vi "weightSerialRead_LoadCell_Fixed_S.vi"(9 "VISA resource name":refnum<visa-resource-name>="COM5") -> (1 "Boolean":bool=TRUE, 2 "Current Weight":string)   [LabVIEW 2019]
uses:
  Program Files (x86)/National Instruments/LabVIEW 2019/examples/Instrument IO/Serial/support/Serial - Settings.ctl
  Program Files (x86)/National Instruments/LabVIEW 2019/examples/Instrument IO/Serial/support/Serial - XON-XOFF Characters.ctl
  Program Files (x86)/National Instruments/LabVIEW 2019/examples/Instrument IO/Serial/support/Serial - ASCII Characters.ctl
  <vilib>/Instr/_visa.llb/VISA Configure Serial Port (Instr).vi
panel:
  in  "Termination Character":u8=10 format="%.0x"
  in  "End Write on Termination Character?":bool=TRUE
  in  "XON/XOFF Characters":T1={"XON"=enum."DC1", "XOFF"=enum."DC3"}
  in  "Serial Settings":T3={"baud rate"=9600, "data bits"=8, "parity"=enum."None", "stop bits"=10, "flow control"=0} {"flow control" items=["None"=0, "XON/XOFF"=1, "RTS/CTS"=2, "DTR/DSR"=4]; "stop bits" items=["1.0"=10, "1.5"=15, "2.0"=20]; "data bits" min=5 max=8 step=1; "baud rate" items=["75"=75, "110"=110, "134"=134, "150"=150, "300"=300, "600"=600, "1200"=1200, "1800"=1800, "2400"=2400, "4800"=4800, "7200"=7200, "9600"=9600, "14400"=14400, "19200"=19200, "28800"=28800, "38400"=38400, "56000"=56000, "57600"=57600, "115200"=115200, "128000"=128000, "230400"=230400]}
  in  "End Read on Termination Character?":bool=TRUE
  in  "Read Count":u32=1000
  out "number":dbl
  in  "Command":string="*IDN?"
  in  "Read":bool=TRUE
  in  "Stop":bool
  in  "Write":bool
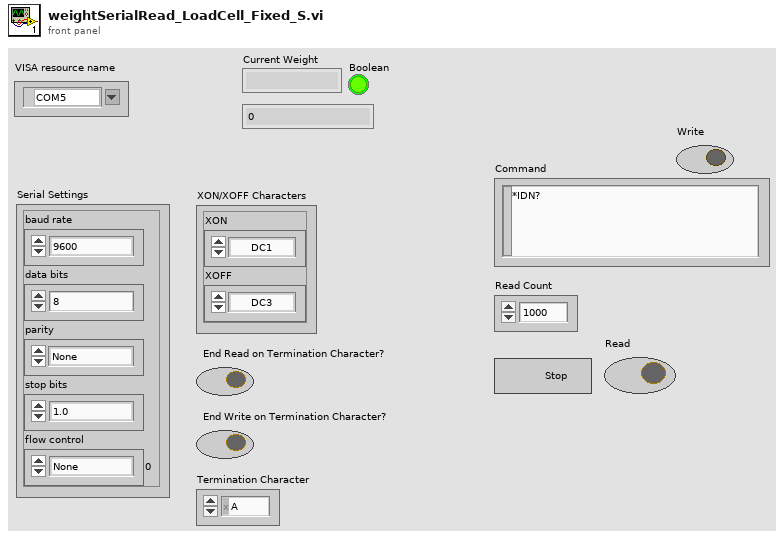
[diagram p1: front panel]
types:
  T1 = typedef "Serial - XON-XOFF Characters.ctl" = cluster{"XON":T2, "XOFF":T2}
  T2 = typedef "Serial - ASCII Characters.ctl" = enum16{"NUL", "SOH", "STX", "ETX", "EOT", "ENQ", "ACK", "BEL", "BS", "HT", "LF", "VT", "FF", "CR", "SO", "SI", "DLE", "DC1", "DC2", "DC3", "DC4", "NAK", "SYN", "ETB", "CAN", "EM", "SUB", "ESC", "FS", "GS", "RS", "US", "SP", "!", "\"", "#", "$", "%", "&", "'", "(", ")", "*", "+", ",", "- (-)", ".", "/", "0", "1", "2", "3", "4", "5", "6", "7", "8", "9", ":", ";", "<", "=", ">", "?", "@", "A", "B", "C", "D", "E", "F", "G", "H", "I", "J", "K", "L", "M", "N", "O", "P", "Q", "R", "S", "T", "U", "V", "W", "X", "Y", "Z", "[", "\\", "]", "^", "_", "`", "a", "b", "c", "d", "e", "f", "g", "h", "i", "j", "k", "l", "m", "n", "o", "p", "q", "r", "s", "t", "u", "v", "w", "x", "y", "z", "{", "|", "}", "~"}
  T3 = typedef "Serial - Settings.ctl" = cluster{"baud rate":u32, "data bits":u16, "parity":enum16{"None", "Odd", "Even", "Mark", "Space"}, "stop bits":u16, "flow control":u16}
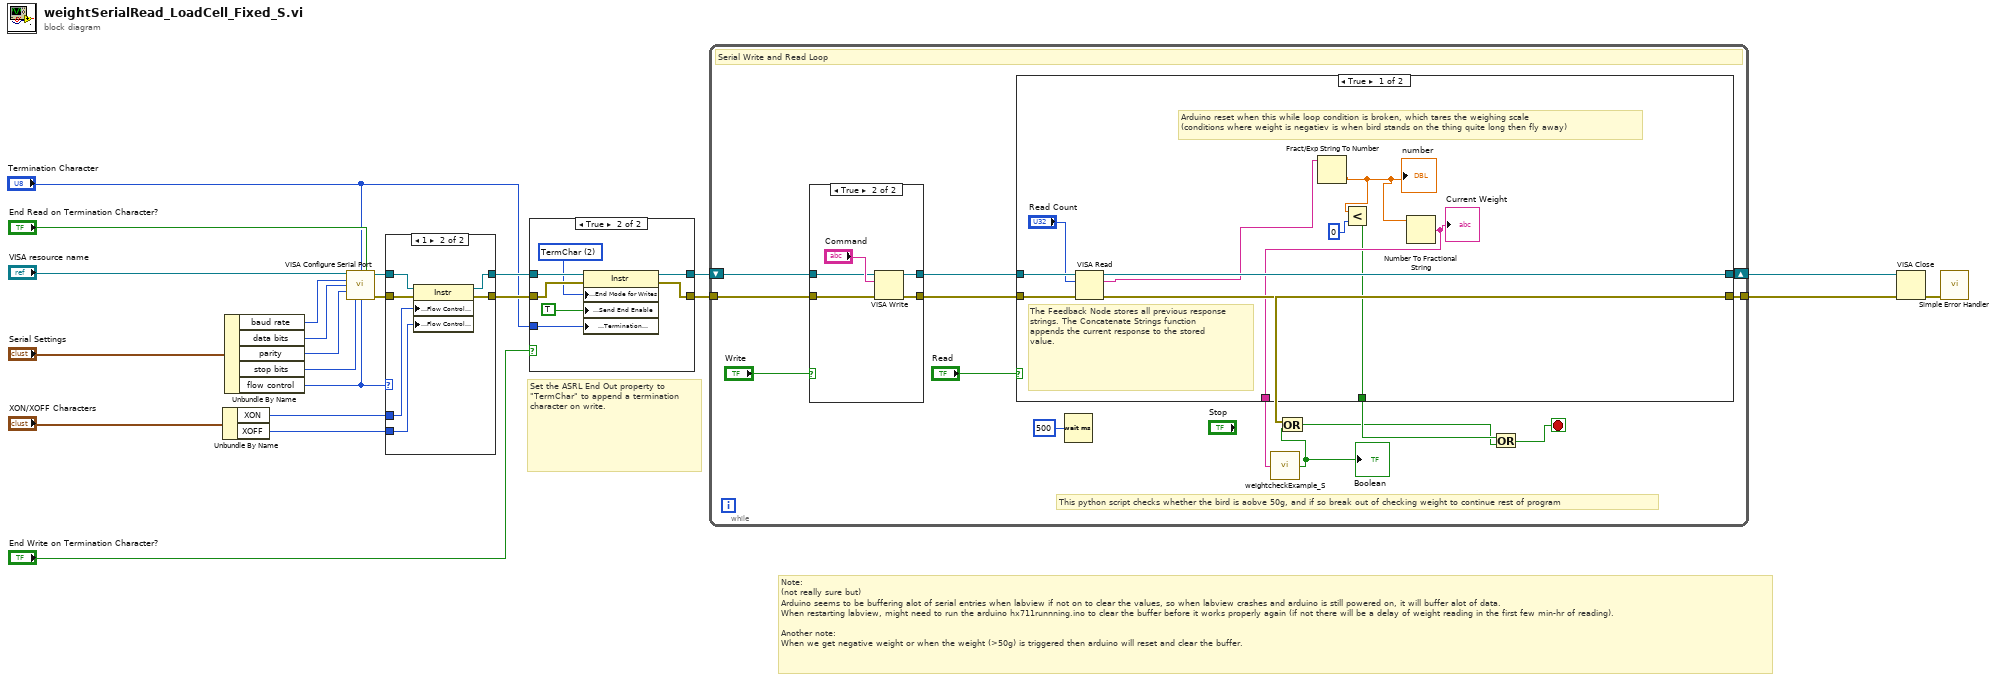
[diagram p0: block diagram]
diagram:
  # "Note: \n(not really sure but) \nArduino seems to be buffering alot of serial entries when labview if not on to clear the values, so when labview crashes and arduino is still powered on, it will buffer alot of data.\nWhen restarting labview, might need to run the arduino hx711runnning.ino to clear the buffer before it works properly again (if not there will be a delay of weight reading in the first few min-hr of reading).\n\nAnother note:\nWhen we get negative weight or when the weight (>50g) is triggered then arduino will reset and clear the buffer."
  # "Set the ASRL End Out property to \"TermChar\" to append a termination character on write."
  n1 = Unbundle By Name("XON/XOFF Characters") -> ("XON"=w8:T2, "XOFF"=w7:T2)
  n2 = Unbundle By Name("Serial Settings") -> ("baud rate"=w15:u32, "data bits"=w16:u16, "parity"=w17:enum16{"None", "Odd", "Even", "Mark", "Space"}, "stop bits"=w18:u16, "flow control"=w9:u16)
  n3 = call-poly "VISA Configure Serial Port"("VISA resource name"="VISA resource name", "termination char\n(0xA = '\\n' = LF)"="Termination Character", "Enable Termination\nChar (T)"="End Read on Termination Character?", "baud rate (9600)"=w15, "data bits (8)"=w16, "parity (0:none)"=w17, "stop bits (10: 1 bit)"=w18, "flow control (0:none)"=w9) -> ("VISA resource name out"=w19:refnum<visa-resource-name>, "error out"=w20:errorcluster)  [unwired: 2 in, 4 out]
  n4 = case shown="1" w9 {
    tunnel: [w23 w30] -> w6
    tunnel: [w24 w29] -> w4
    tunnel: w20 -> [w23 w28]
    tunnel: w19 -> [w24 w27]
    tunnel: w8 -> [_ w26]
    tunnel: w7 -> [_ w25]
    frame Default {
    }
    frame 1 {
      n5 = property class="Instr"(reference=w27, error in=w28, "Serial Settings:Flow Control XON Character"=w26, "Serial Settings:Flow Control XOFF Character"=w25) -> (reference out=w29:refnum<visa-resource-name>, error out=w30:errorcluster)
    }
  }
  n6 = case shown="True" "End Write on Termination Character?" {
    tunnel: w4 -> [w31 w39]
    tunnel: w6 -> [w32 w38]
    tunnel: [w31 w37] -> w3
    tunnel: [w32 w36] -> w5
    tunnel: "Termination Character" -> [_ w34]
    frame False {
    }
    frame True {
      w35 = u16 2 items=["None", "LastBit", "TermChar", "Break"] ("Serial Settings:Serial End Mode for Writes")
      n7 = property class="Instr"(reference=w39, error in=w38, "Serial Settings:End Mode for Writes"=w35, "Message Based Settings:Send End Enable"=TRUE, "Message Based Settings:Termination Character"=w34) -> (reference out=w37:refnum<visa-resource-name>, error out=w36:errorcluster)
    }
  }
  n8 = while {
    shift-right: [w53] -> w10
    shift-left: w3 -> [w52]
    tunnel: w5 -> [w51]
    tunnel: [w46] -> w11
    stop <- w40 stop-if-true
    # "This python script checks whether the bird is aobve 50g, and if so break out of checking weight to continue rest of program"
    # "Serial Write and Read Loop"
    n9 = case shown="True" "Write" {
      tunnel: w52 -> [w55 w59]
      tunnel: w51 -> [w54 w58]
      tunnel: [w55 w57] -> w50
      tunnel: [w54 w56] -> w49
      frame False {
      }
      frame True {
        n10 = VISA Write(VISA resource name=w59, write buffer="Command", error in (no error)=w58) -> (VISA resource name out=w57:refnum<visa-resource-name>, error out=w56:errorcluster)  [unwired: 1 out]
      }
    }
    n11 = case shown="True" "Read" {
      tunnel: [w68 w72] -> w53
      tunnel: w50 -> [w70 w72]
      tunnel: [w66 w71] -> w46
      tunnel: w49 -> [w69 w71]
      tunnel: [w64 _] -> w44
      tunnel: [w61 _] -> w42
      frame True {
        # "Arduino reset when this while loop condition is broken, which tares the weighing scale \n(conditions where weight is negatiev is when bird stands on the thing quite long then fly away)"
        # "The Feedback Node stores all previous response strings. The Concatenate Strings function appends the current response to the stored value."
        n12 = VISA Read(VISA resource name=w70, byte count="Read Count", error in (no error)=w69) -> (VISA resource name out=w68:refnum<visa-resource-name>, read buffer=w65:string, error out=w66:errorcluster)  [unwired: 1 out]
        n13 = Fract/Exp String To Number(string=w65) -> (number=w63:dbl)  [unwired: 3 in, 1 out]
        "number" <- w63
        n14 = Less?(x=w63, y=0) -> (x < y?=w61:bool)
        n15 = Number To Fractional String(number=w63) -> (F-format string=w64:string)  [unwired: 3 in]
        "Current Weight" <- w64
      }
      frame False {
      }
    }
    n16 = Wait (ms)(milliseconds to wait=u32 500) -> ()  [unwired: 1 out]
    n17 = call "weightcheckExample_S.vi"("weight"=w44) -> ("Boolean"=w43:bool)
    "Boolean" <- w43
    n18 = Or(x=w46, y=w43) -> (x .or. y?=w41:bool)
    n19 = Or(x=w42, y=w41) -> (x .or. y?=w40:bool)
  }
  n20 = VISA Close(VISA resource name=w10, error in (no error)=w11) -> (error out=w12:errorcluster)
  n21 = call <vilib>:"Simple Error Handler.vi"("error in (no error)"=w12) -> ()  [unwired: 1 in, 8 out]
